vi "axis_to_bool.vi"(1 "in":dbl) -> (0 "out":bool)   [LabVIEW 2020]
panel:
  in  "threshold":dbl=0.07
  # "Outputs true if the input squared is greater than the threshold"
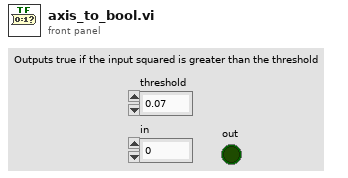
[diagram p1: front panel]
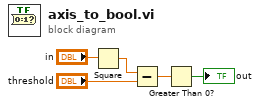
[diagram p0: block diagram]
diagram:
  n1 = Square(x="in") -> (x^2=w4:dbl)
  n2 = Subtract(x=w4, y="threshold") -> (x-y=w2:dbl)
  n3 = Greater Than 0?(x=w2) -> (x > 0?=→"out":bool)
